vi "Get database list.vi"(0 "InfluxDB in":refnum<class "InfluxDB Client.lvclass">, 11 "error in (no error)":errorcluster) -> (4 "InfluxDB out":refnum<class "InfluxDB Client.lvclass">, 6 "Database names":string[](array[string]), 15 "error out":errorcluster)   [LabVIEW 2013, in "InfluxDB Client.lvclass"]
doc: "Gets a list of available databases."
uses:
  InfluxDB Client.lvclass
  InfluxDB Client.lvclass/InfluxDB Client.ctl
  <vilib>/LVH/i3 JSON/JSON Parsing/Get Array Value at Index Files/Get Array Value at Index - Object.vi
  <vilib>/LVH/i3 JSON/JSON Parsing/Get Object Parameter Files/Get Object Parameter - String.vi
  <vilib>/httpClient/LabVIEWHTTPClient.lvlib
  <vilib>/LVH/i3 JSON/i3-json.lvlib
panel:
  out "Status":string
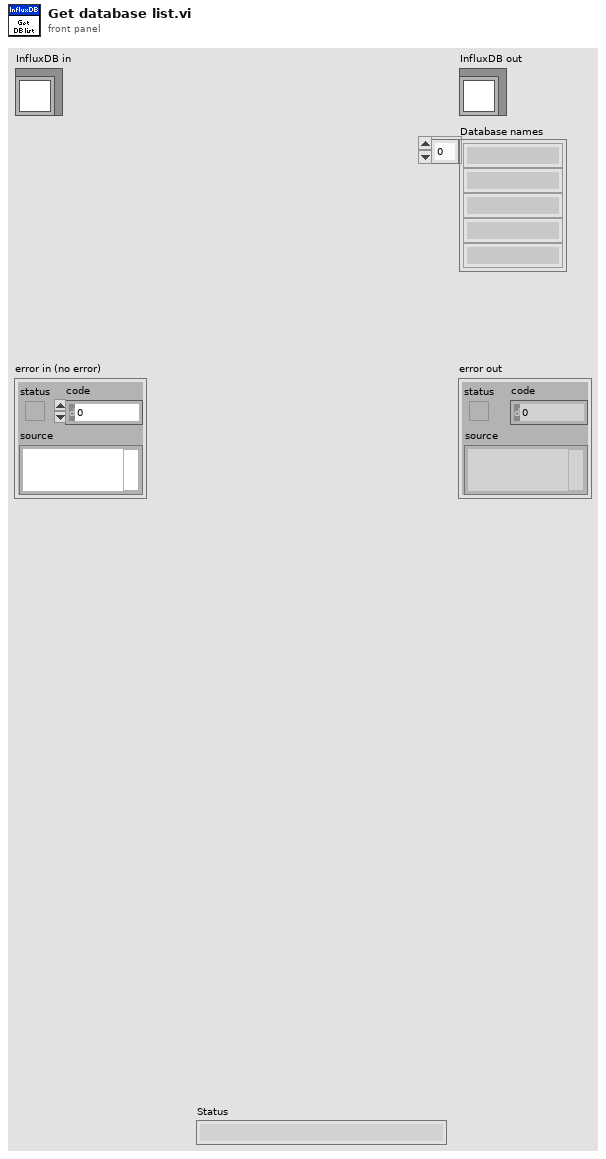
[diagram p1: front panel]
types:
  T1 = typedef "LabVIEWHTTPClient.lvlib/ClientHandle.ctl" = refnum<k1>
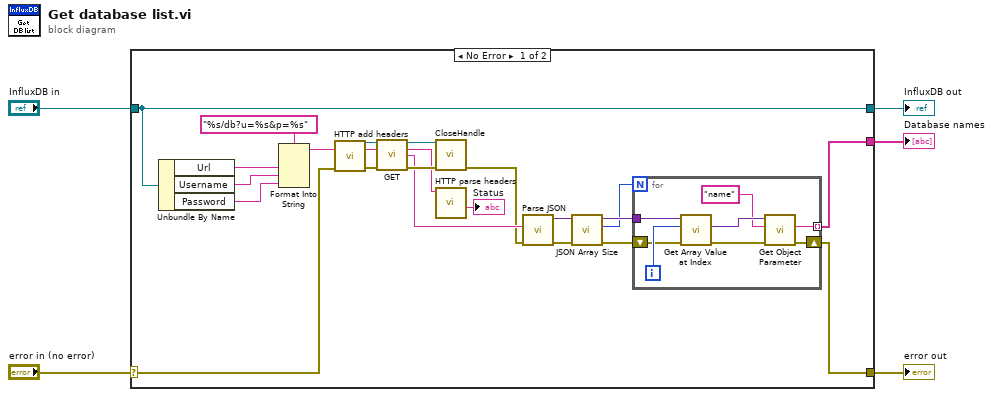
[diagram p0: block diagram]
diagram:
  n1 = case shown="No Error" "error in (no error)" {
    selector: "error in (no error)" -> [w17 w37]
    tunnel: [w7 w37] -> w4
    tunnel: [w27 w36] -> w2
    tunnel: "InfluxDB in" -> [w27 w36]
    tunnel: [w11 _] -> w1
    frame No Error {
      n2 = Unbundle By Name(w27) -> ("Url"=w25:string, "Username"=w19:string, "Password"=w18:string)
      n3 = Format Into String(format string="%s/db?u=%s&p=%s" ("url"), w25, w19, w18) -> (resulting string=w22:string)  [unwired: 2 in, 1 out]
      n4 = call "HTTP add headers.vi"("error in (no error)"=w17) -> ("client handle out"=w15:T1, "error out"=w16:errorcluster)  [unwired: 13 in]
      n5 = call <vilib>:"GET.vi"("client handle"=w15, "url"=w22, "error in (no error)"=w16) -> ("client handle out"=w24:T1, "headers"=w21:string, "body"=w10:string, "error out"=w23:errorcluster)  [unwired: 9 in]
      n6 = call <vilib>:"CloseHandle.vi"("client handle"=w24, "error in (no error)"=w23) -> ("error out"=w6:errorcluster)  [unwired: 13 in]
      n7 = call "HTTP parse headers.vi"("HTTP headers"=w21) -> ("Status"=→"Status":string)  [unwired: 8 in, 2 out]
      n8 = call <vilib>:"Parse JSON.vi"("error in (no error)"=w6, "JSON String"=w10) -> ("error out"=w9:errorcluster, "JSON Tree"=w12:variant)  [unwired: 6 in, 2 out]
      n9 = call <vilib>:"JSON Array Size.vi"("error in (no error)"=w9, "JSON Tree In (JSON Array)"=w12) -> ("error out"=w8:errorcluster, "Array Size"=w13:i32, "JSON Tree Passthrough (JSON Array)"=w14:variant)  [unwired: 7 in]
      n10 = for {
        N: w13 -> [_]
        tunnel: w14 -> [w35]
        tunnel: [w31] -> w11 mode=indexing
        shift-right: [w28] -> w7
        shift-left: w8 -> [w30]
        i -> [w34]
        n11 = call-poly <vilib>:"Get Array Value at Index.vi"("error in (no error)"=w30, "Index"=w34, "JSON Tree In (JSON Array)"=w35) -> ("error out"=w29:errorcluster, "JSON Object"=w33:variant)  [unwired: 5 in, 2 out]
        n12 = call-poly <vilib>:"Get Object Parameter.vi"("error in (no error)"=w29, "Parameter Name"="name", "JSON Tree In (JSON Object)"=w33) -> ("error out"=w28:errorcluster, "String Value"=w31:string)  [unwired: 5 in, 2 out]
      }
    }
    frame Error {
    }
  }
  "error out" <- w4
  "InfluxDB out" <- w2
  "Database names" <- w1
